vi "PH_PowerUnit_BaseClass.Set State SM to GUI.vi"(0 "i ref in":refnum<vi>, 2 "State SM":string, 5 "error in (no error)":errorcluster) -> (14 "i ref out":refnum<vi>, 19 "error out":errorcluster)   [LabVIEW 2014, in "PH_PowerUnit_BaseClass.lvlib"]
doc: "This VI writes the state of the SM to the GUI element."
uses:
  PH_PowerUnit_BaseClass.lvlib
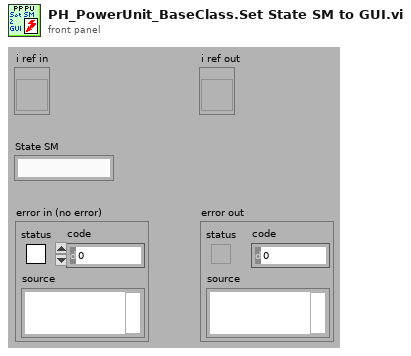
[diagram p1: front panel]
types:
  T1 = typedef "PH_PowerUnit_BaseClass.lvlib/PH_PowerUnit_BaseClass.SM States.ctl" = enum16{".", "Stand by", "Switch PU on", "Configure", "Set Default Voltage", "Set STANDBY", "Set READY", "Wait for Shot Cmd", "Open Dump Rods", "Open Ross Relais", "Close Ross Relais", "Switch PSU on", "Switch PSU off", "Charge", "Switch GD Channel on", "Close Dump Rods", "Rods-TO", "RR-TO", "PSU-TO", "Trigger-TO"}
  T2 = typedef "PH_PowerUnit_BaseClass.lvlib/PH_PowerUnit_BaseClass.i attribute.ctl" = cluster{"Constructor finished":bool, "PU":cluster{"In use":bool, "Service ID in use":i32, "GUI Ref":refnum<vi>}, "Enabling":cluster{"State":T3, "GUI Ref":refnum<vi>}, "Timing":cluster{"Last Shot":dbl, "Time between Shots [Sec]":dbl, "Waiting Time over?":bool, "Service ID Waiting Time":i32, "GUI Ref":refnum<vi>, "Instance":cluster{"Status":T4, "linked?":bool, "GUI Ref":refnum<vi>}}, "Sequencer":cluster{"SM State":string, "GUI Ref":refnum<vi>, "linked":bool}, "Subscribed Trendmssgs":cluster{"Tagname":string, "Status":T4, "linked?":bool, "Shot Condition":T4, "GUI Ref":refnum<vi>}[], "PP PU":T5, "Default Voltage (V)":dbl, "GUI Refs":T6, "PSDB data":cluster{"Shot Voltage [V]":dbl, "State TO SM":T1, "Write 2 early":bool}, "State TO SM":T1}
  T3 = typedef "PH_SystemInformation.lvlib/PH_SystemInformationEnabling State.ctl" = i32
  T4 = typedef "PH_StatusHandler.lvlib/PH_StatusHandler.Status.ctl" = i16
  T5 = typedef "PH_PP_Common.lvlib/PH_PP_Common.PUs.ctl" = enum16{"no Info", "PA-19mm-1", "PA-19mm-2", "PA-45mm-PILC", "PA-45mm-MAIN", "MA-PU-1", "MA-PU-2", "MA-PU-3", "MA-PU-4", "MA-PU-5", "MA-PU-6", "MA-FR", "MA-PILC", "PA-45mm-DP"}
  T6 = typedef "PH_PowerUnit_BaseClass.lvlib/PH_PowerUnit_BaseClass.GUI Refs.ctl" = cluster{"Delete Inst":refnum<vi>, "State TO SM":refnum<vi>, "State SM":refnum<vi>, "Fire":refnum<vi>}
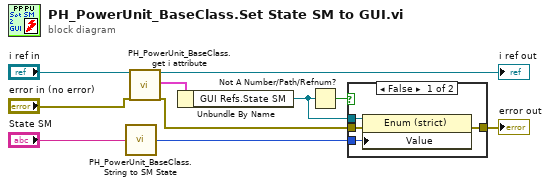
[diagram p0: block diagram]
diagram:
  n1 = call "PH_PowerUnit_BaseClass.String to SM State.vi"("SM State String"="State SM") -> ("SM State"=w1:T1)
  n2 = call "PH_PowerUnit_BaseClass.get i attribute.vi"("i ref in"="i ref in", "error in (no error)"="error in (no error)") -> ("i ref out"=→"i ref out":refnum<vi>, "i attribute"=w7:T2, "error out"=w5:errorcluster)  [unwired: 15 in]
  n3 = Unbundle By Name(w7) -> ("GUI Refs.State SM"=w4:refnum<vi>)
  n4 = Not A Number/Path/Refnum?(number/path/refnum=w4) -> (NaN/Path/Refnum?=w3:bool)
  n5 = case shown="False" w3 {
    tunnel: [w14 w15] -> w6
    tunnel: w4 -> [w13 _]
    tunnel: w5 -> [w12 w15]
    tunnel: w1 -> [w11 _]
    frame False {
      n6 = property class="Enum (strict)"(reference=w13, error in=w12, "Value"=w11) -> (error out=w14:errorcluster)  [unwired: 1 out]
    }
    frame True {
    }
  }
  "error out" <- w6
